vi "1-10.vi"() -> ()   [LabVIEW 2022 SP3]
panel:
  out "布尔":bool
  in  "数值 2":dbl
  in  "数值":dbl
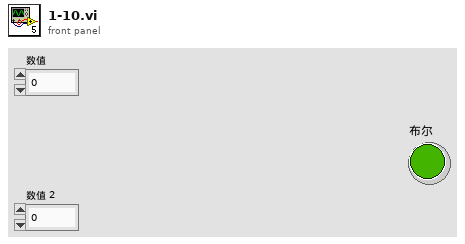
[diagram p1: front panel]
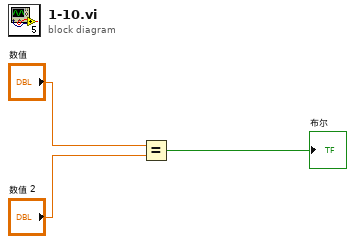
[diagram p0: block diagram]
diagram:
  n1 = Equal?(x="数值", y="数值 2") -> (x = y?=→"布尔":bool)
